vi "GetAttributeViInt32.vi"(8 "error in (no error)":errorcluster {"code" format="%.0x"}, 9 "AttributeID":u32(ring)=1150002 items=["CHANNEL_AVERAGING_FACTOR"=1150002, "CHANNEL_COUNT"=1150185, "CHANNEL_MEASUREMENT_COUNT"=1150105, "CHANNEL_MEASUREMENT_ELECTRICAL_DELAY_MEDIUM"=1150178, "CHANNEL_MEASUREMENT_ELECTRICAL_DELAY_UNITS"=1150175, "CHANNEL_MEASUREMENT_FORMAT"=1150014, "CHANNEL_MEASUREMENT_LIMIT_NUMBER"=1150020, "CHANNEL_MEASUREMENT_MARKER_COUNT"=1150104, "CHANNEL_MEASUREMENT_NUMBER"=1150163, "CHANNEL_MEASUREMENT_TIME_DOMAIN_GATING_SHAPE"=1150140, "CHANNEL_MEASUREMENT_TIME_DOMAIN_GATING_TYPE"=1150144, "CHANNEL_MEASUREMENT_TIME_DOMAIN_PARAMETERS"=1150137, "CHANNEL_MEASUREMENT_TIME_DOMAIN_TRANSFORM_MODE"=1150147, "CHANNEL_MEASUREMENT_TRACE_MATH"=1150017, "CHANNEL_NUMBER"=1150006, "CHANNEL_POINTS"=1150007, "CHANNEL_SWEEP_MODE"=1150009, "CHANNEL_SWEEP_TYPE"=1150012, "CHANNEL_TRIGGER_MODE"=1150013, "GUIDED_CALIBRATION__CALIBRATION_STEP_ITERATION_COUNT"=1150158, "GUIDED_CALIBRATION_CALIBRATION_STEP_COUNT"=1150106, "GUIDED_CALIBRATION_CALIBRATION_STEP_MINIMUM_ITERATIONS"=1150159, "GUIDED_CALIBRATION_CALIBRATION_STEP_NUMBER"=1150160, "GUIDED_CALIBRATION_STEP_COUNT"=1150118, "MAXIMUM_NUMBER_OF_CHANNELS"=1150168, "MAXIMUM_NUMBER_OF_POINTS"=1150167, "STATUS_SERIAL_POLL"=1150037, "SYSTEM_TIME_OUT_MILLISECONDS"=1150040, "TEST_PORT_COUNT"=1150166, "TRIGGER_SOURCE"=1150042, "WINDOW_COUNT"=1150108, "WINDOW_NUMBER"=1150130, "WINDOW_SIZE"=1150133, "WINDOW_TABLE"=1150134], 10 "RepCapIdentifier":string, 11 "instrument handle":refnum<k15>) -> (0 "error out":errorcluster {"code" format="%.0x"}, 2 "AttributeValue":i32, 3 "instrument handle out":refnum<k15>)   [LabVIEW 2014, in "Agilent NA.lvlib"]
doc: "Gets an Int32 attribute from the instrument driver.\nThe following Attributes are supported:\n\nCHANNEL_AVERAGING_FACTOR\nCHANNEL_COUNT\nCHANNEL_MEASUREMENT_COUNT\nCHANNEL_MEASUREMENT_ELECTRICAL_DELAY_MEDIUM\nCHANNEL_MEASUREMENT_ELECTRICAL_DELAY_UNITS\nCHANNEL_MEASUREMENT_FORMAT\nCHANNEL_MEASUREMENT_LIMIT_NUMBER\nCHANNEL_MEASUREMENT_MARKER_COUNT\nCHANNEL_MEASUREMENT_NUMBER\nCHANNEL_MEASUREMENT_TIME_DOMAIN_GATING_SHAPE\nCHANNEL_MEASUREMENT_TIME_DOMAIN_GATING_TYPE\nCHANNEL_MEASUREMENT_TIME_DOMAIN_PARAMETERS\nCHANNEL_MEASUREMENT_TIME_DOMAIN_TRANSFORM_MODE\nCHANNEL_MEASUREMENT_TRACE_MATH\nCHANNEL_NUMBER\nCHANNEL_POINTS\nCHANNEL_SWEEP_MODE\nCHANNEL_SWEEP_TYPE\nCHANNEL_TRIGGER_MODE\nGUIDED_CALIBRATION__CALIBRATION_STEP_ITERATION_COUNT\nGUIDED_CALIBRATION_CALIBRATION_STEP_COUNT\nGUIDED_CALIBRATION_CALIBRATION_STEP_MINIMUM_ITERATIONS\nGUIDED_CALIBRATION_CALIBRATION_STEP_NUMBER\nGUIDED_CALIBRATION_STEP_COUNT\nMAXIMUM_NUMBER_OF_CHANNELS\nMAXIMUM_NUMBER_OF_POINTS\nSTATUS_SERIAL_POLL\nSYSTEM_TIME_OUT_MILLISECONDS\nTEST_PORT_COUNT\nTRIGGER_SOURCE\nWINDOW_COUNT\nWINDOW_NUMBER\nWINDOW_SIZE\nWINDOW_TABLE"
uses:
  Agilent NA.lvlib
  AgNA.dll
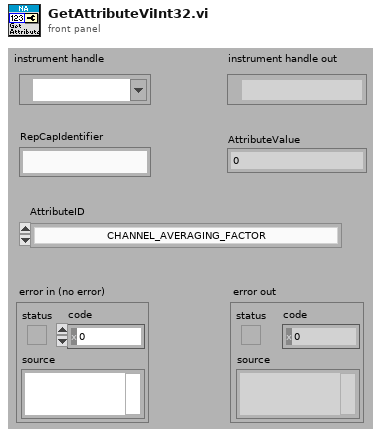
[diagram p1: front panel]
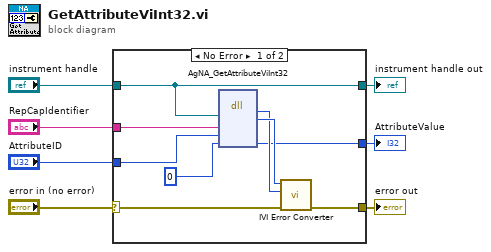
[diagram p0: block diagram]
diagram:
  n1 = case shown="No Error" "error in (no error)" {
    selector: "error in (no error)" -> [w14 w18]
    tunnel: [w13 w18] -> w7
    tunnel: "RepCapIdentifier" -> [w12 _]
    tunnel: "AttributeID" -> [w11 _]
    tunnel: [w9 _] -> w3
    tunnel: [w8 w17] -> w2
    tunnel: "instrument handle" -> [w8 w17]
    frame No Error {
      n2 = dll-call lib="AgNA**.dll" fn="AgNA_GetAttributeViInt32"("Vi"=w8, "RepCapIdentifier"=w12, "AttributeID"=w11, "AttributeValue"=0) -> ("return type"=w15:i32, "Vi"=w16:u32, "AttributeValue"=w9:i32)  [unwired: 5 in, 2 out]
      n3 = call "IVI Error Converter.vi"("error in (no error)"=w14, "IVI error code (0)"=w15, "instrument handle"=w16) -> ("error out"=w13:errorcluster)  [unwired: 7 in, 1 out]
    }
    frame Error {
    }
  }
  "error out" <- w7
  "instrument handle out" <- w2
  "AttributeValue" <- w3
